vi "Motor SetupV2.vi"(8 "error in (no error)":errorcluster) -> (0 "error out":errorcluster, 3 "mecanum steering frame out":refnum<class "NI_Robotics_Mecanum Steering Frame.lvclass">)   [LabVIEW 2012]
uses:
  <vilib>/robotics/Steering/Mecanum Steering Frame/NI_Robotics_Mecanum Steering Frame.lvclass
  <vilib>/robotics/Steering/Wheel/Wheel Parameters.ctl
  <vilib>/robotics/Steering/Wheel/Rotation Direction.ctl
  <vilib>/robotics/Steering/Mecanum Wheel/Roller Orientation.ctl
  <vilib>/robotics/Steering/Mecanum Wheel/Create Mecanum Wheel.vi
  <vilib>/robotics/Steering/Mecanum Steering Frame/Create Mecanum Steering Frame.vi
  <vilib>/robotics/Steering/Wheel/NI_Robotics_Wheel.lvclass
  <vilib>/robotics/Steering/Mecanum Wheel/NI_Robotics_Mecanum Wheel.lvclass
  <vilib>/robotics/Steering/Steering Frame/NI_Robotics_Steering Frame.lvclass
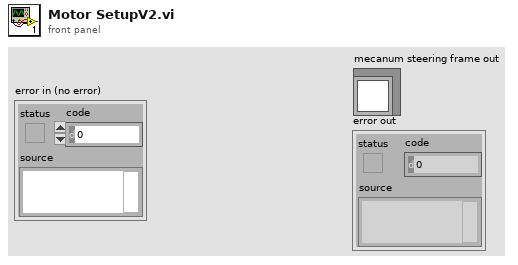
[diagram p1: front panel]
types:
  T1 = typedef "NI_Robotics_Mecanum Wheel.lvclass/Roller Orientation.ctl" = u16
  T2 = typedef "NI_Robotics_Wheel.lvclass/Wheel Parameters.ctl" = cluster{"wheel radius":dbl, "gear ratio":dbl, "forward rotation direction":T3}
  T3 = typedef "NI_Robotics_Wheel.lvclass/Rotation Direction.ctl" = u16
  T4 = cluster{"mecanum wheel out":refnum<class "NI_Robotics_Mecanum Wheel.lvclass">, "mecanum wheel out":refnum<class "NI_Robotics_Mecanum Wheel.lvclass">, "mecanum wheel out":refnum<class "NI_Robotics_Mecanum Wheel.lvclass">, "mecanum wheel out":refnum<class "NI_Robotics_Mecanum Wheel.lvclass">}
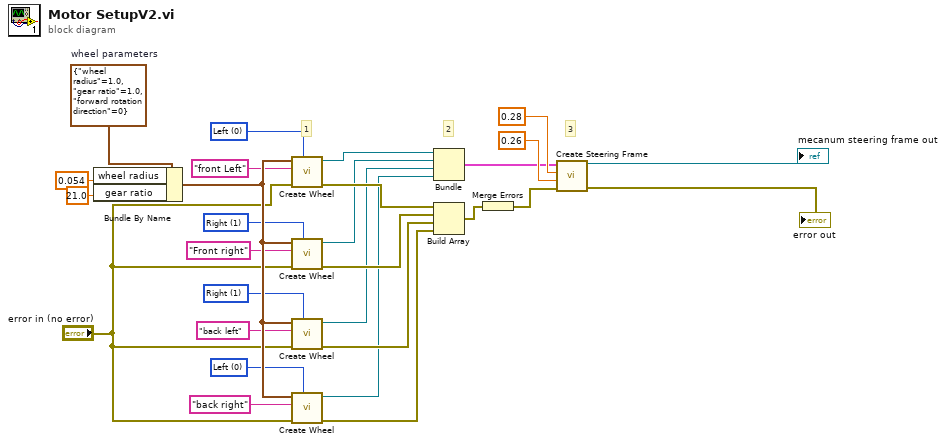
[diagram p0: block diagram]
diagram:
  w5 = T1 0 items=["Left", "Right"] ("roller orientation")
  w6 = T1 1 items=["Left", "Right"] ("roller orientation")
  w7 = T1 1 items=["Left", "Right"] ("roller orientation")
  w8 = T1 0 items=["Left", "Right"] ("roller orientation")
  w13 = T2 {"wheel radius"=1.0, "gear ratio"=1.0, "forward rotation direction"=0}  # wheel parameters
  # "3"
  # "2"
  # "1"
  n1 = Bundle By Name(cluster=w13, "wheel radius"=0.054, "gear ratio"=21.0) -> (w12:T2)
  n2 = call-poly <vilib>:"Create Wheel.vi"("roller orientation"=w8, "error in (no error)"="error in (no error)", "wheel name"="front Left", "wheel parameters"=w12) -> ("error out"=w23:errorcluster, "mecanum wheel out"=w16:refnum<class "NI_Robotics_Mecanum Wheel.lvclass">)  [unwired: 6 in]
  n3 = call-poly <vilib>:"Create Wheel.vi"("roller orientation"=w7, "error in (no error)"="error in (no error)", "wheel name"="Front right", "wheel parameters"=w12) -> ("error out"=w24:errorcluster, "mecanum wheel out"=w17:refnum<class "NI_Robotics_Mecanum Wheel.lvclass">)  [unwired: 6 in]
  n4 = call-poly <vilib>:"Create Wheel.vi"("roller orientation"=w6, "error in (no error)"="error in (no error)", "wheel name"="back left", "wheel parameters"=w12) -> ("error out"=w25:errorcluster, "mecanum wheel out"=w18:refnum<class "NI_Robotics_Mecanum Wheel.lvclass">)  [unwired: 6 in]
  n5 = call-poly <vilib>:"Create Wheel.vi"("roller orientation"=w5, "error in (no error)"="error in (no error)", "wheel name"="back right", "wheel parameters"=w12) -> ("error out"=w27:errorcluster, "mecanum wheel out"=w19:refnum<class "NI_Robotics_Mecanum Wheel.lvclass">)  [unwired: 6 in]
  n6 = Bundle("mecanum wheel out"=w16, "mecanum wheel out"=w17, "mecanum wheel out"=w18, "mecanum wheel out"=w19) -> (w20:T4)  [unwired: 1 in]
  n7 = Build Array(w23, w24, w25, w27) -> (w26:errorcluster[])
  n8 = Merge Errors(w26) -> (w28:errorcluster)
  n9 = call-poly <vilib>:"Create Steering Frame.vi"("error in (no error)"=w28, "wheel separation length"=0.26, "wheel separation width"=0.28, "wheels"=w20) -> ("error out"=→"error out":errorcluster, "mecanum steering frame out"=→"mecanum steering frame out":refnum<class "NI_Robotics_Mecanum Steering Frame.lvclass">)  [unwired: 6 in]
